vi "FlowMeterStubSatu.vi"(6 "Graph in":cluster{dbl[], dbl[]}, 7 "Index":i32, 8 "error in":errorcluster, 9 "Length":i32=250, 11 "ON":bool) -> (0 "error out":errorcluster, 2 "Values":cluster{dbl[], dbl[]})   [LabVIEW 2012]
uses:
  GlobalVariables/CalibrationState.vi
  GlobalVariables/CalibrationVolumes.vi
  GlobalVariables/Samples.vi
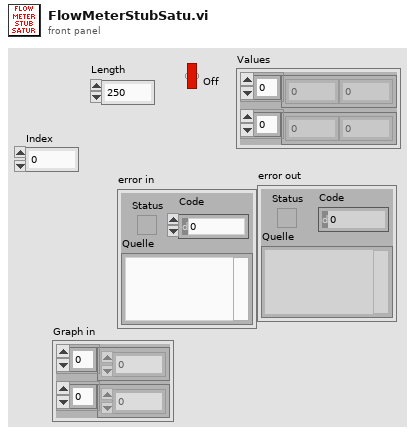
[diagram p1: front panel]
types:
  T1 = cluster{"Pressure":cluster{"TimeSamples":dbl[], "PressureSamples":dbl[]}, "Flow":cluster{"TimeSamples":dbl[], "FlowSamples":dbl[]}}
  T2 = cluster{"CalibrationVolumes":dbl[], "SetName":string}[]
  T3 = cluster{bool, "CalibrationStep":u32, "PressureCons":dbl[], "PressureMes":dbl[], "Weights":bool[], "CalibrationCaptor":u32}
  T4 = cluster{"TimeSamples":dbl[], "FlowSamples":dbl[]}
  T5 = cluster{"TimeSamples":dbl[], "PressureSamples":dbl[]}
  T6 = cluster{"Pressure":cluster{"TimeSamples":dbl[], "PressureSamples":dbl[]}, cluster{"TimeSamples":dbl[], "FlowSamples":dbl[]}}
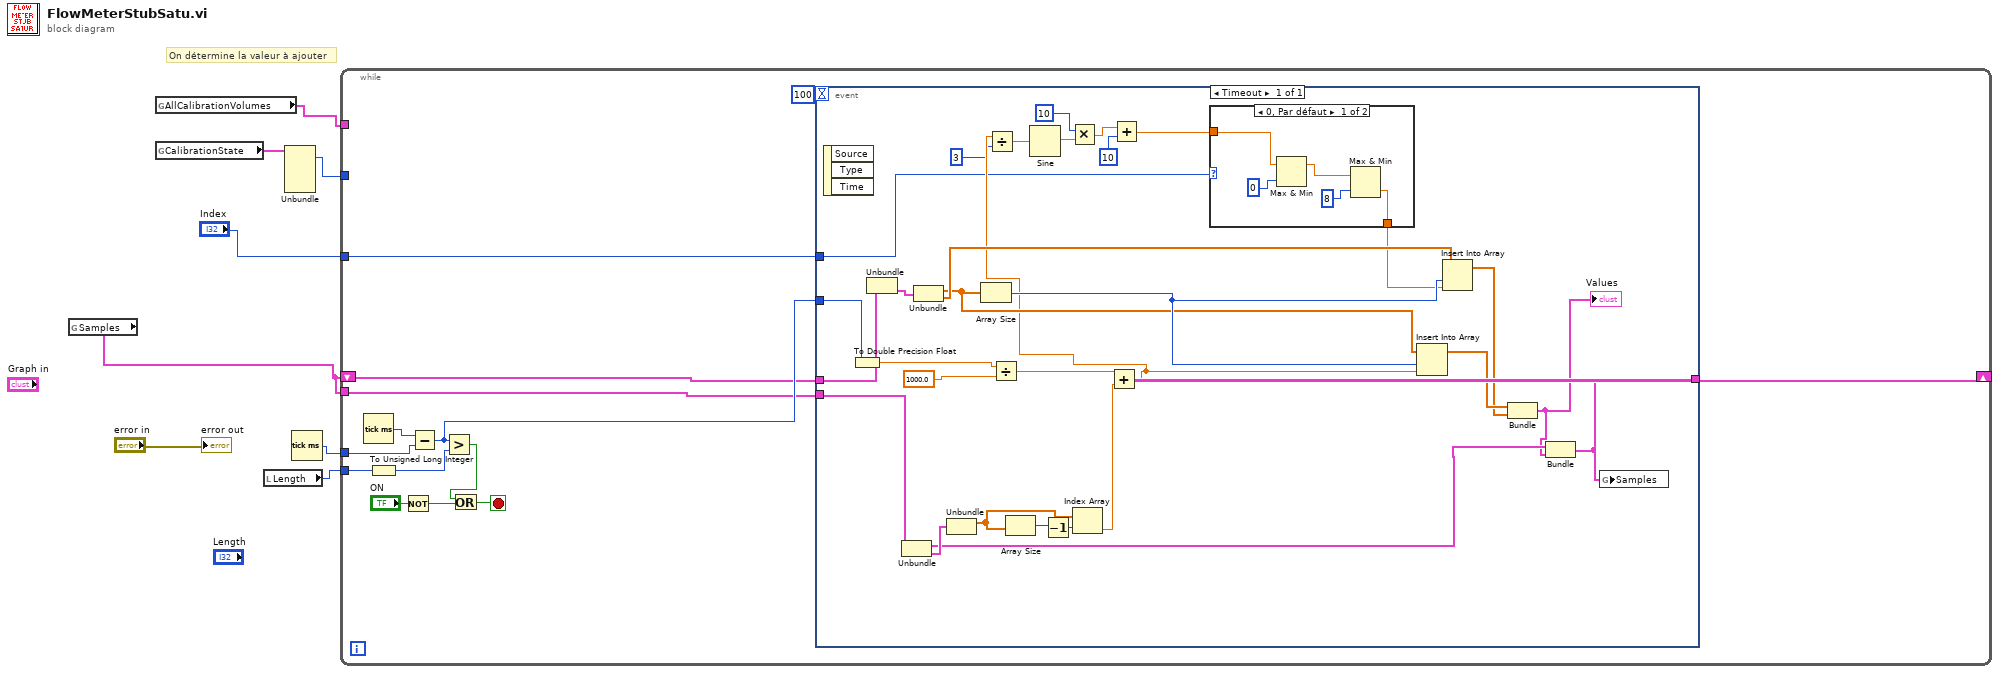
[diagram p0: block diagram]
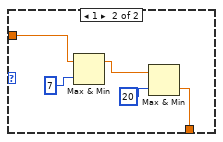
[diagram p2: hidden frame]
diagram:
  # "On détermine la valeur à ajouter"
  n1 = global read "Samples.vi" "Samples"() -> (w2:T1)
  n2 = global read "CalibrationVolumes.vi" "AllCalibrationVolumes"() -> (w4:T2)
  n3 = global read "CalibrationState.vi" "CalibrationState"() -> (w5:T3)
  n4 = local read "Length"() -> (w7:i32)
  n5 = Unbundle(w5) -> ("CalibrationStep"=w3:u32)  [unwired: 5 out]
  n6 = Tick Count (ms)() -> (millisecond timer value=w8:u32)
  n7 = while {
    tunnel: w8 -> [w18]
    tunnel: w7 -> [w13]
    shift-right: [w11] -> _
    shift-left: w2 -> [w14]
    tunnel: w4 -> [_]
    tunnel: w3 -> [_]
    tunnel: w2 -> [w10]
    tunnel: "Index" -> [w9]
    stop <- w20 stop-if-true
    n8 = Tick Count (ms)() -> (millisecond timer value=w19:u32)
    n9 = To Unsigned Long Integer(number=w13) -> (unsigned 32bit integer=w12:u32)
    n10 = Not(x="ON") -> (.not. x?=w21:bool)
    n11 = Subtract(x=w19, y=w18) -> (x-y=w15:u32)
    n12 = Greater?(x=w15, y=w12) -> (0:w17:bool)
    n13 = Or(x=w17, y=w21) -> (x .or. y?=w20:bool)
    n14 = event shown="[0] Timeout" {
      selector: _ -> [_]
      dyn-events: _ -> [_]
      timeout: 100 -> [_]
      tunnel: w15 -> [w48]
      tunnel: w14 -> [w45]
      tunnel: [w37] -> w11
      tunnel: w10 -> [w44]
      tunnel: w9 -> [w29]
      event Timeout {
        n15 = event-data() -> ()  [unwired: 1 in, 3 out]
        n16 = To Double Precision Float(number=w48) -> (double precision float=w47:dbl)
        n17 = Unbundle(w45) -> ("Flow"=w26:T4)  [unwired: 1 out]
        n18 = Unbundle(w44) -> ("Pressure"=w24:T5, "Flow"=w25:T4)
        n19 = Unbundle(w26) -> ("TimeSamples"=w38:dbl[], "FlowSamples"=w39:dbl[])
        n20 = Unbundle(w25) -> ("TimeSamples"=w40:dbl[])  [unwired: 1 out]
        n21 = Array Size(array=w38) -> (size(s)=w43:i32)
        n22 = Divide(x=w47, y=1000.0) -> (x/y=w49:dbl)
        n23 = Array Size(array=w40) -> (size(s)=w52:i32)
        n24 = Decrement(x=w52) -> (x-1=w51:i32)
        n25 = Index Array(array=w40, index=w51) -> (element=w46:dbl)
        n26 = Add(x=w49, y=w46) -> (x+y=w32:dbl)
        n27 = Divide(x=w32, y=3) -> (x/y=w31:dbl)
        n28 = Sine(x=w31) -> (sin(x)=w35:dbl)
        n29 = Multiply(x=10, y=w35) -> (x*y=w34:dbl)
        n30 = Add(x=w34, y=10) -> (x+y=w28:dbl)
        n31 = case shown="0, Par défaut" w29 {
          tunnel: w28 -> [w57 w59]
          tunnel: [w53 w58] -> w27
          frame 0, Default {
            n32 = Max & Min(x=w57, y=0) -> (max(x,y)=w54:dbl)  [unwired: 1 out]
            n33 = Max & Min(x=w54, y=8) -> (min(x,y)=w53:dbl)  [unwired: 1 out]
          }
          frame 1 {
            n34 = Max & Min(x=w59, y=7) -> (max(x,y)=w60:dbl)  [unwired: 1 out]
            n35 = Max & Min(x=w60, y=20) -> (min(x,y)=w58:dbl)  [unwired: 1 out]
          }
        }
        n36 = Insert Into Array(array=w38, index=w43, new element=w32) -> (w42:dbl[])
        n37 = Insert Into Array(array=w39, index=w43, new element=w27) -> (w41:dbl[])
        n38 = Bundle("TimeSamples"=w42, "FlowSamples"=w41) -> (w23:T4)  [unwired: 1 in]
        "Values" <- w23
        n39 = Bundle("Pressure"=w24, w23) -> (w37:T6)  [unwired: 1 in]
        n40 = global write "Samples.vi" "Samples"(w37) -> ()
      }
    }
  }
  "error out" <- "error in"
